vi "camera tests.vi"() -> ()   [LabVIEW 2021, in "Test VIs.lvclass"]
uses:
  Test VIs.lvclass
  Classes/Controller/Camera/QR Code Reader/QR Code Reader.lvclass
  C:/Users/HEP/Documents/GitHub/Gantry/UCSB-Gantry-HEP-main/Classes/Controller/Camera/Camera.lvclass
  Classes/Controller/Camera/Edmund Optics/Edmund Optics.lvclass
  Classes/Controller/Camera/Camera.lvclass
  Classes/Controller/Motion/Motion.lvclass
  Classes/Controller/Motion/A3200/A3200.lvclass
panel:
  out "XYZTheta Out":dbl[](array[numeric])
  in  "done?":bool
  out "Image 2":T1(plugin-control)
  out "Image":T1(plugin-control)
  in  "Switch to little camera":bool
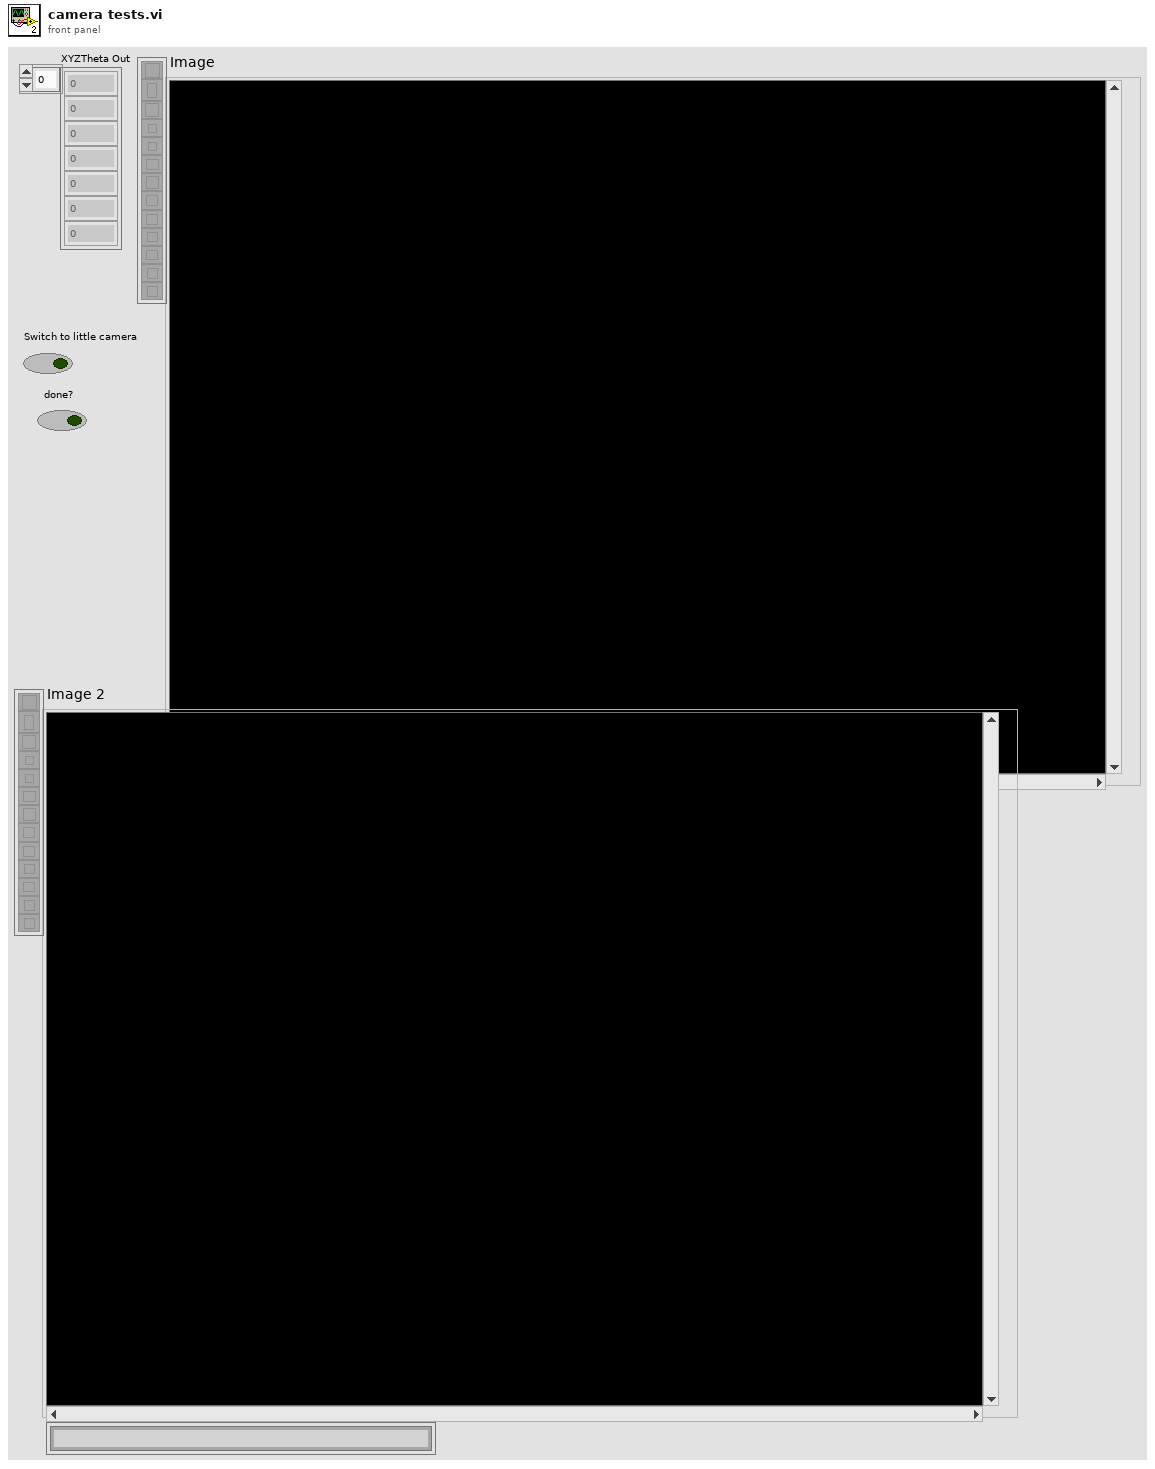
[diagram p1: front panel]
types:
  T1 = typedef "IMAQ Image.ctl" = refnum<image>
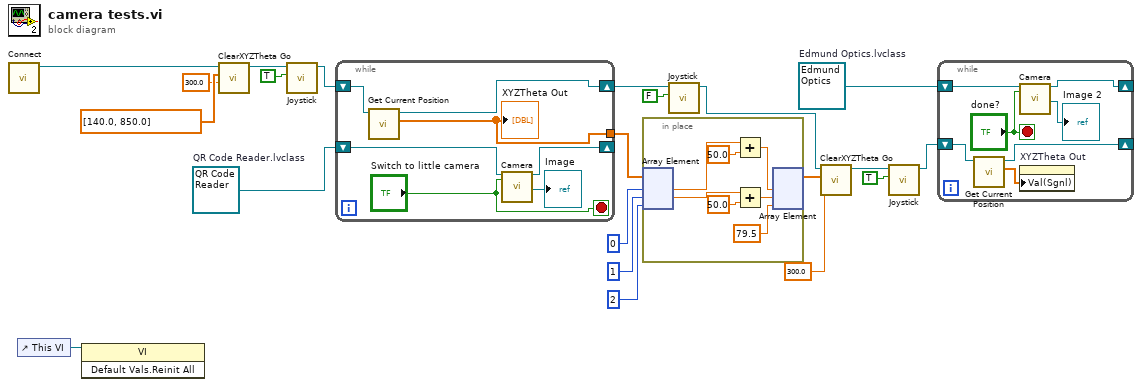
[diagram p0: block diagram]
diagram:
  w20 = refnum<class "Edmund Optics.lvclass"> refnum  # Edmund Optics.lvclass
  w21 = refnum<class "QR Code Reader.lvclass"> refnum  # QR Code Reader.lvclass
  n1 = call "Connect.vi"() -> ("Gantry 3"=w6:refnum<k24>)  [unwired: 10 in, 1 out]
  n2 = control-ref of="This VI"() -> (w7:refnum<vi>)
  n3 = invoke class="VI" method="Default Vals.Reinit All"(reference=w7) -> ()  [unwired: 2 in, 3 out]
  n4 = call "ClearXYZTheta Go.vi"("Speed"=300.0, "XYZTheta In"=dbl[] [140.0, 850.0], "Gantry In"=w6) -> ("Gantry Out"=w4:refnum<k24>)  [unwired: 6 in, 2 out]
  n5 = call "Joystick.vi"("Joystick"=TRUE, "Gantry In"=w4) -> ("Gantry Out"=w12:refnum<k24>)  [unwired: 8 in, 1 out]
  n6 = while {
    shift-right: [w27] -> _
    shift-left: w21 -> [w28]
    shift-right: [w23] -> w10
    shift-left: w12 -> [w24]
    tunnel: [w22] -> w14
    stop <- "Switch to little camera" stop-if-true
    n7 = call "Get Current Position.vi"("Gantry In"=w24) -> ("XYZTheta Out"=w22:dbl[], "Gantry Out"=w23:refnum<k24>)  [unwired: 8 in, 1 out]
    "XYZTheta Out" <- w22
    n8 = call "Camera.vi"("Camera in"=w28, "Stop"="Switch to little camera") -> ("Camera out"=w27:refnum<class "QR Code Reader.lvclass">, "Image"=→"Image":T1)  [unwired: 10 in, 6 out]
  }
  n9 = in-place {
    n10 = in-place-array #1(w14, 0, 1, 2) -> (w35:dbl, w32:dbl)  [unwired: 1 out]
    n11 = Add(x=w35, y=50.0) -> (x+y=w34:dbl)
    n12 = Add(x=w32, y=50.0) -> (x+y=w33:dbl)
    n13 = in-place-array #1(w34, w33, 79.5 ("element")) -> (w13:dbl[])  [unwired: 3 out]
  }
  n14 = call "Joystick.vi"("Joystick"=FALSE, "Gantry In"=w10) -> ("Gantry Out"=w9:refnum<k24>)  [unwired: 8 in, 1 out]
  n15 = call "ClearXYZTheta Go.vi"("Speed"=300.0, "XYZTheta In"=w13, "Gantry In"=w9) -> ("Gantry Out"=w19:refnum<k24>)  [unwired: 6 in, 2 out]
  n16 = call "Joystick.vi"("Joystick"=TRUE, "Gantry In"=w19) -> ("Gantry Out"=w18:refnum<k24>)  [unwired: 8 in, 1 out]
  n17 = while {
    shift-right: [w41] -> _
    shift-left: w20 -> [w42]
    shift-right: [w37] -> _
    shift-left: w18 -> [w38]
    stop <- "done?" stop-if-true
    n18 = call "Get Current Position.vi"("Gantry In"=w38) -> ("XYZTheta Out"=w36:dbl[], "Gantry Out"=w37:refnum<k24>)  [unwired: 8 in, 1 out]
    n19 = call "Camera.vi"("Camera in"=w42, "Stop"="done?") -> ("Camera out"=w41:refnum<class "Edmund Optics.lvclass">, "Image"=→"Image 2":T1)  [unwired: 10 in, 6 out]
    n20 = property on="XYZTheta Out" class="Arr (strict)"("Val(Sgnl)"=w36) -> ()  [unwired: 2 in, 2 out]
  }
